vi "Lift_Function.vi"(6 "Low Range":T1, 7 "High Range":T2, 9 "Input Cluster":T3={"Level 5"=TRUE, "Level 4"=TRUE, "Level 3"=TRUE, "Level 2"=TRUE, "Level 1"=FALSE}, 10 "MotorControlDevRef":T4={"DeviceStatus"={"status"=FALSE, "code"=0, "source"=""}, "Type"=enum."PWM", "PWM"={"Controller"=enum."Controller 1", "PWM Channel"=enum."Invalid", "DeadBand"={"Name"="", "maxPositivePwm"=0, "minPositivePwm"=0, "centerPwm"=0, "maxNegativePwm"=0, "minNegativePwm"=0, "angularRange"=0}}, "CAN"={"Device Number"=0, "Control Mode"=enum."Percent VBus", "Semaphore"=refnum, "Max Vout"=12.0, "TalonSRX Control Mode"=enum."Percent VBus"}, "Invert"=FALSE, "TransformRef"=refnum, "InvTransformRef"=refnum}, 11 "EncoderDevRef":T13={"DevStatus"={"status"=FALSE, "code"=0, "source"=""}, "EncoderIndex"=enum."Invalid", "CounterIndex"=enum."Ctr 1", "DistancePerCount"=2.0, "Decoding Type"=enum."4x"}) -> (3 "Output Cluster":T3)   [LabVIEW 2014]
uses:
  <vilib>/Rock Robotics/SystemInterfaces/Encoder/FPGA_EncoderIdx.ctl
  <vilib>/Rock Robotics/WPI/Encoder/WPI_EncoderType.ctl
  <vilib>/Rock Robotics/SystemInterfaces/Counter/FPGA_CounterCtrSystemIndex.ctl
  <vilib>/Rock Robotics/WPI/Encoder/WPI_EncoderDevRef.ctl
  <vilib>/Rock Robotics/WPI/MotorControl/WPI_MotorControlDeviceRef.ctl
  <vilib>/Rock Robotics/WPI/PWM/WPI_PWMTransform_ConPane.ctl
  <vilib>/Rock Robotics/SystemInterfaces/Typedef/FPGA_TypedefDigitalModule.ctl
  <vilib>/Rock Robotics/SystemInterfaces/DIO/FPGA_DIOPWMChannel.ctl
  <vilib>/Rock Robotics/WPI/PWM/WPI_PWMDeadband.ctl
  <vilib>/Rock Robotics/WPI/CAN/Jaguar/SubVIs/WPI_CANJaguar_ControlMode.ctl
  <vilib>/Rock Robotics/WPI/CAN/TalonSRX/WPI_CANTalonSRX_APIControlMode.ctl
  <vilib>/Rock Robotics/WPI/MotorControl/WPI_MotorControlType.ctl
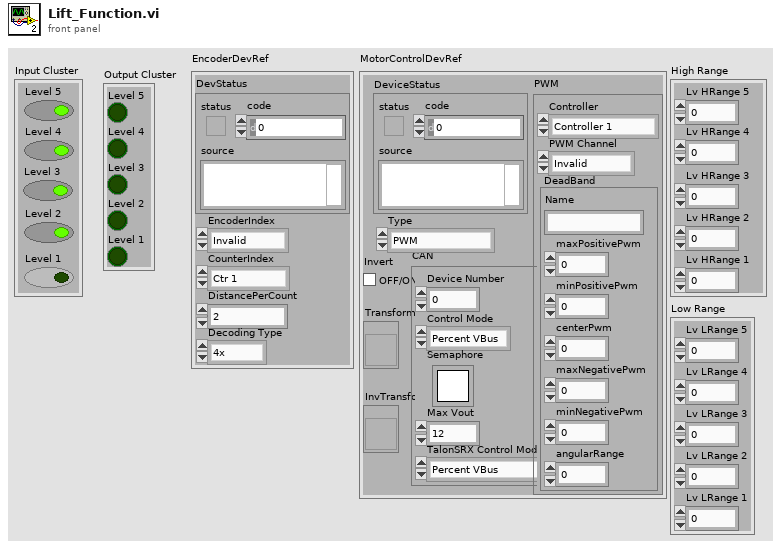
[diagram p1: front panel]
types:
  T1 = cluster{"Lv LRange 1":dbl, "Lv LRange 2":dbl, "Lv LRange 3":dbl, "Lv LRange 4":dbl, "Lv LRange 5":dbl}
  T2 = cluster{"Lv HRange 5":dbl, "Lv HRange 4":dbl, "Lv HRange 3":dbl, "Lv HRange 2":dbl, "Lv HRange 1":dbl}
  T3 = cluster{"Level 5":bool, "Level 4":bool, "Level 3":bool, "Level 2":bool, "Level 1":bool}
  T4 = typedef "WPI_MotorControlDeviceRef.ctl" = cluster{"DeviceStatus":errorcluster, "Type":T5, "PWM":cluster{"Controller":T6, "PWM Channel":T7, "DeadBand":T8}, "CAN":cluster{"Device Number":u8, "Control Mode":T9, "Semaphore":T10, "Max Vout":dbl, "TalonSRX Control Mode":T11}, "Invert":bool, "TransformRef":T12, "InvTransformRef":T12}
  T5 = typedef "WPI_MotorControlType.ctl" = enum16{"PWM", "CAN", "CANTalonSRX"}
  T6 = typedef "FPGA_TypedefDigitalModule.ctl" = enum16{"Controller 1"}
  T7 = typedef "FPGA_DIOPWMChannel.ctl" = enum8{"PWM 0", "PWM 1", "PWM 2", "PWM 3", "PWM 4", "PWM 5", "PWM 6", "PWM 7", "PWM 8", "PWM 9", "PWM MXP 0", "PWM MXP 1", "PWM MXP 2", "PWM MXP 3", "PWM MXP 4", "PWM MXP 5", "PWM MXP 6", "PWM MXP 7", "PWM MXP 8", "PWM MXP 9", "Invalid"}
  T8 = typedef "WPI_PWMDeadband.ctl" = cluster{"Name":string, "maxPositivePwm":i32, "minPositivePwm":i32, "centerPwm":i32, "maxNegativePwm":i32, "minNegativePwm":i32, "angularRange":u16}
  T9 = typedef "WPI_CANJaguar_ControlMode.ctl" = enum8{"Percent VBus", "Current", "Speed", "Position", "Voltage"}
  T10 = typedef "Semaphore RefNum" = refnum<k1>
  T11 = typedef "WPI_CANTalonSRX_APIControlMode.ctl" = enum8{"Percent VBus", "Speed", "Position", "Slave", "Unchanged / Invalid"}
  T12 = typedef "WPI_PWMTransform_ConPane.ctl" = refnum<vi>
  T13 = typedef "WPI_EncoderDevRef.ctl" = cluster{"DevStatus":errorcluster, "EncoderIndex":T14, "CounterIndex":T15, "DistancePerCount":dbl, "Decoding Type":T16}
  T14 = typedef "FPGA_EncoderIdx.ctl" = enum8{"Enc 0", "Enc 1", "Enc 2", "Enc 3", "Enc 4", "Enc 5", "Enc 6", "Enc 7", "Invalid"}
  T15 = typedef "FPGA_CounterCtrSystemIndex.ctl" = enum8{"Ctr 0", "Ctr 1", "Ctr 2", "Ctr 3", "Ctr 4", "Ctr 5", "Ctr 6", "Ctr 7", "Invalid"}
  T16 = typedef "WPI_EncoderType.ctl" = enum16{"1x", "2x", "4x"}
  T17 = cluster{"Level":bool, "Level":bool, "Level":bool, "Level":bool, "Level":bool}
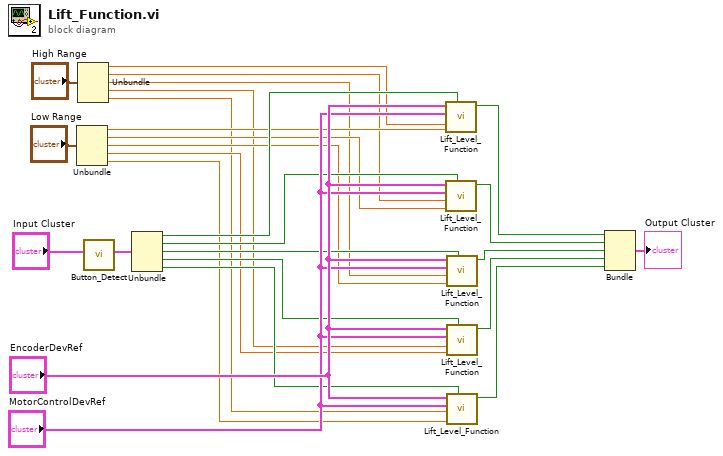
[diagram p0: block diagram]
diagram:
  n1 = Unbundle("Low Range") -> ("Lv LRange 1"=w9:dbl, "Lv LRange 2"=w8:dbl, "Lv LRange 3"=w6:dbl, "Lv LRange 4"=w4:dbl, "Lv LRange 5"=w2:dbl)
  n2 = Unbundle("High Range") -> ("Lv HRange 5"=w10:dbl, "Lv HRange 4"=w7:dbl, "Lv HRange 3"=w1:dbl, "Lv HRange 2"=w5:dbl, "Lv HRange 1"=w3:dbl)
  n3 = call "Button_Detect.vi"("Input Cluster"="Input Cluster") -> ("Output Cluster"=w19:T3)  [unwired: 10 in]
  n4 = Unbundle(w19) -> ("Level 5"=w18:bool, "Level 4"=w17:bool, "Level 3"=w16:bool, "Level 2"=w15:bool, "Level 1"=w14:bool)
  n5 = call "Lift_Level_Function.vi"("Level"=w18, "upper limit"=w9, "lower Limit"=w10, "MotorControlDevRef"="MotorControlDevRef", "EncoderDevRef"="EncoderDevRef") -> ("Level"=w25:bool)  [unwired: 6 in]
  n6 = call "Lift_Level_Function.vi"("Level"=w17, "upper limit"=w8, "lower Limit"=w7, "MotorControlDevRef"="MotorControlDevRef", "EncoderDevRef"="EncoderDevRef") -> ("Level"=w24:bool)  [unwired: 6 in]
  n7 = call "Lift_Level_Function.vi"("Level"=w16, "upper limit"=w6, "lower Limit"=w1, "MotorControlDevRef"="MotorControlDevRef", "EncoderDevRef"="EncoderDevRef") -> ("Level"=w23:bool)  [unwired: 6 in]
  n8 = call "Lift_Level_Function.vi"("Level"=w15, "upper limit"=w4, "lower Limit"=w5, "MotorControlDevRef"="MotorControlDevRef", "EncoderDevRef"="EncoderDevRef") -> ("Level"=w22:bool)  [unwired: 6 in]
  n9 = call "Lift_Level_Function.vi"("Level"=w14, "upper limit"=w2, "lower Limit"=w3, "MotorControlDevRef"="MotorControlDevRef", "EncoderDevRef"="EncoderDevRef") -> ("Level"=w21:bool)  [unwired: 6 in]
  n10 = Bundle("Level"=w25, "Level"=w24, "Level"=w23, "Level"=w22, "Level"=w21) -> (→"Output Cluster":T17)  [unwired: 1 in]
